vi "Init_HovaCAL Controls.vi"(8 "Fehler (Eingang, kein Fehler)":errorcluster, 10 "Refs Cluster":T1, 11 "Info Cluster":T2) -> (0 "Fehler (Ausgang)":errorcluster)   [LabVIEW 2020, in "EPA 1065.lvlib" / "HovaCAL Interference verificaton.lvlib"]
uses:
  HovaCAL Interference verificaton.lvlib
  Linearisierung V2/Gasteiler/HovaCAL_Interface/Controls/Info Cluster.ctl
  Linearisierung V2/Gasteiler/HovaCAL_Interface/Controls/Controls.lvlib
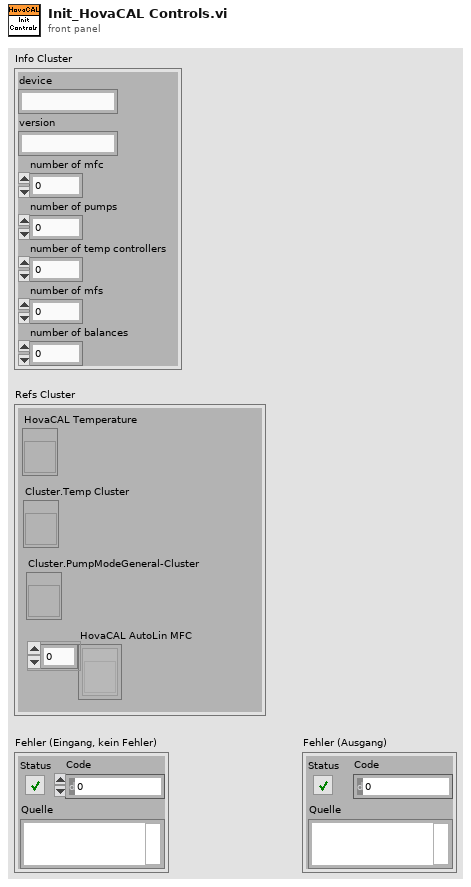
[diagram p1: front panel]
types:
  T1 = cluster{"HovaCAL Temperature":refnum<vi>, "Cluster.Temp Cluster":refnum<vi>, "Cluster.PumpModeGeneral-Cluster":refnum<vi>, "HovaCAL AutoLin MFC":refnum<vi>[]}
  T2 = typedef "Linearisierung v2.lvlib/Gasteiler.lvlib/HovaCAL_Interface.lvlib/Controls.lvlib/Info Cluster.ctl" = cluster{"device":string, "version":string, "number of mfc":i32, "number of pumps":i32, "number of temp controllers":i32, "number of mfs":i32, "number of balances":i32}
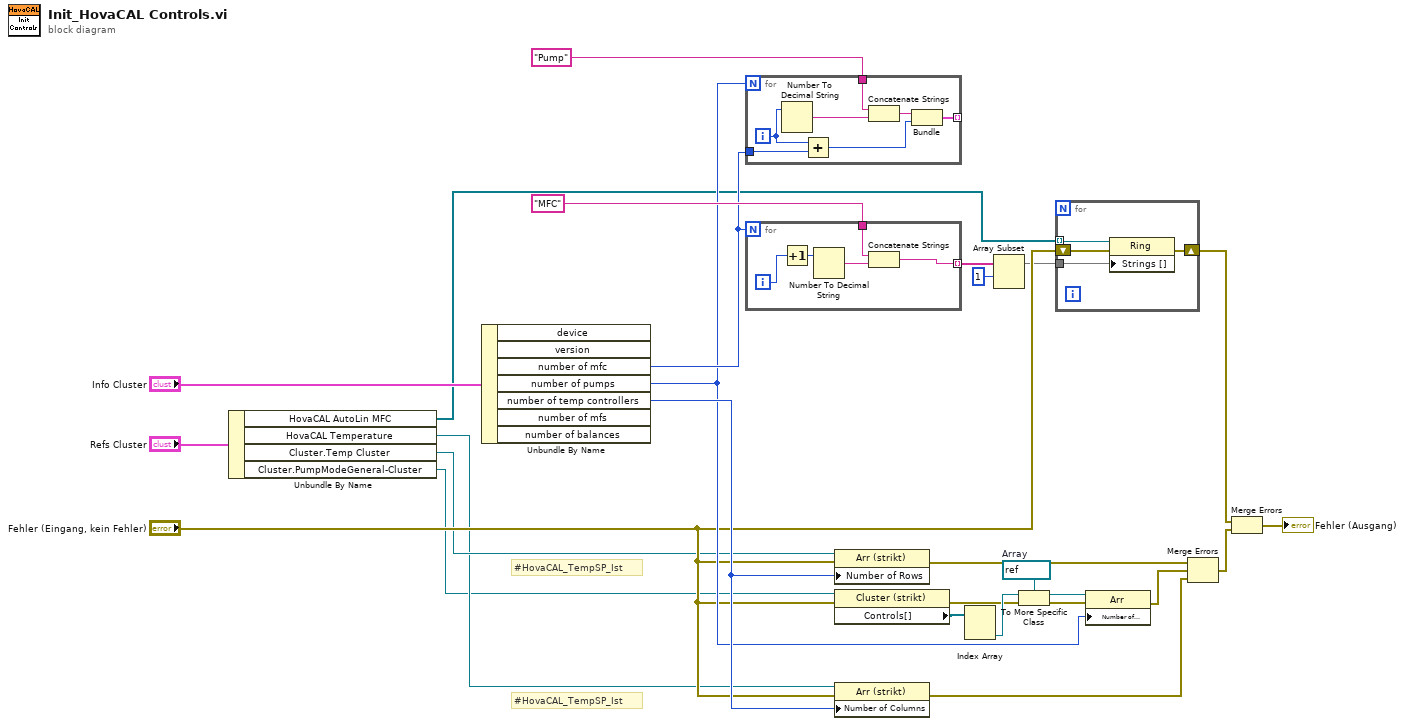
[diagram p0: block diagram]
diagram:
  w20 = refnum<vi> refnum  # Array
  # "#HovaCAL_TempSP_Ist"
  # "#HovaCAL_TempSP_Ist"
  n1 = Unbundle By Name("Refs Cluster") -> ("HovaCAL AutoLin MFC"=w5:refnum<vi>[], "HovaCAL Temperature"=w7:refnum<vi>, "Cluster.Temp Cluster"=w8:refnum<vi>, "Cluster.PumpModeGeneral-Cluster"=w6:refnum<vi>)
  n2 = Unbundle By Name("Info Cluster") -> ("number of mfc"=w12:i32, "number of pumps"=w11:i32, "number of temp controllers"=w14:i32)  [unwired: 4 out]
  n3 = for {
    N: w11 -> [_]
    tunnel: [w34] -> _ mode=indexing
    tunnel: "Pump" ("String") -> [w30]
    tunnel: w12 -> [w28]
    i -> [w33]
    n4 = Number To Decimal String(number=w33) -> (decimal integer string=w32:string)  [unwired: 1 in]
    n5 = Add(x=w33, y=w28) -> (x+y=w29:i32)
    n6 = Concatenate Strings(w30, w32) -> (w31:string)
    n7 = Bundle(w31, w29) -> (w34:cluster{string, i32})  [unwired: 1 in]
  }
  n8 = for {
    N: w12 -> [_]
    tunnel: [w35] -> w24 mode=indexing
    tunnel: "MFC" ("String") -> [w37]
    i -> [w39]
    n9 = Increment(x=w39) -> (x+1=w36:i32)
    n10 = Number To Decimal String(number=w36) -> (decimal integer string=w38:string)  [unwired: 1 in]
    n11 = Concatenate Strings(w37, w38) -> (w35:string)
  }
  n12 = property class="Arr (strikt)"(reference=w8, error in="Fehler (Eingang, kein Fehler)", "Number of Rows"=w14) -> (error out=w22:errorcluster)  [unwired: 1 out]
  n13 = property class="Cluster (strikt)"(reference=w6, error in="Fehler (Eingang, kein Fehler)") -> (error out=w17:errorcluster, "Controls[]"=w21:refnum<vi>[])  [unwired: 1 out]
  n14 = property class="Arr (strikt)"(reference=w7, error in="Fehler (Eingang, kein Fehler)", "Number of Columns"=w14) -> (error out=w3:errorcluster)  [unwired: 1 out]
  n15 = Index Array(array=w21) -> (element #2=w19:refnum<vi>)  [unwired: 2 in, 1 out]
  n16 = Array Subset(array=w24, index=1 ("Index")) -> (w2:string[])  [unwired: 1 in]
  n17 = To More Specific Class(target class=w20, reference=w19, error in=w17) -> (specific class reference=w18:refnum<vi>, error out=w16:errorcluster)
  n18 = for {
    tunnel: w2 -> [w40]
    shift-right: [w43] -> w23
    shift-left: "Fehler (Eingang, kein Fehler)" -> [w42]
    tunnel: w5 -> [w41] mode=indexing
    n19 = property class="Ring"(reference=w41, error in=w42, "Strings []"=w40) -> (error out=w43:errorcluster)  [unwired: 1 out]
  }
  n20 = property class="Arr"(reference=w18, error in=w16, "Number of Columns"=w11) -> (error out=w15:errorcluster)  [unwired: 1 out]
  n21 = Merge Errors(w22, w15, w3) -> (w4:errorcluster)
  n22 = Merge Errors(w23, w4) -> (→"Fehler (Ausgang)":errorcluster)
